vi "Execute.vi"(8 "error in":errorcluster, 11 "Filter STEP in":refnum<class "Filter STEP.lvclass">) -> (0 "error out":errorcluster, 1 "Next Step?":bool, 2 "MSG":string, 3 "Filter STEP out":refnum<class "Filter STEP.lvclass">)   [LabVIEW 2014, in "Filter STEP.lvclass"]
uses:
  Filter STEP.lvclass
  <vilib>/ActorFramework/Message Enqueuer/Message Enqueuer.lvclass
  Controller/Messages/Change Filter State/Change Filter State.lvclass
  Controller/Messages/Update Switch State MSG/Update Switch MSG.lvclass/Update Switch MSG.ctl
  <vilib>/ActorFramework/Message Enqueuer/Message Enqueuer.lvclass/Message Enqueuer.ctl
  Controller/Messages/Update Switch State MSG/Write Val.vi
  <vilib>/ActorFramework/Message Priority Queue/Priority Enqueue.vi
  c/exscalabar/steps/SEQ.lvlibp/STEPS/Read Obj.vi
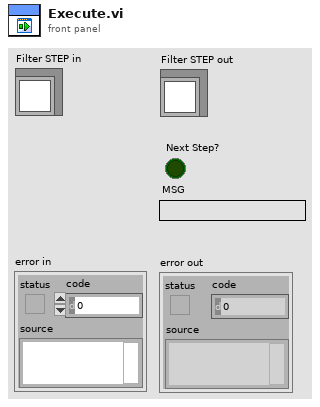
[diagram p1: front panel]
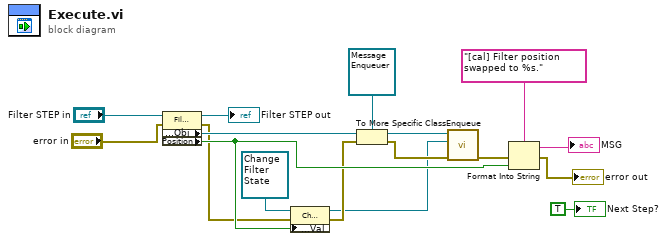
[diagram p0: block diagram]
diagram:
  n1 = property class="Filter"(reference="Filter STEP in", error in="error in") -> (reference out=→"Filter STEP out":refnum<class "Filter STEP.lvclass">, error out=w10:errorcluster, "Accessors:Obj"=w17:refnum<class>, "Position"=w11:bool)
  n2 = property class="Change Filter State MSG"(reference=refnum<class "Change Filter State.lvclass"> refnum ("Controller:Change Filter State MSG"), error in=w10, "Accessors:Val"=w11) -> (reference out=w2:refnum<class "Change Filter State.lvclass">, error out=w9:errorcluster)
  n3 = To More Specific Class(target class=refnum<class "Message Enqueuer.lvclass"> refnum ("Message Enqueuer in"), reference=w17, error in=w9) -> (specific class reference=w14:refnum<class "Message Enqueuer.lvclass">, error out=w15:errorcluster)
  n4 = call <vilib>:"Enqueue.vi"("error in (no error)"=w15, "Message"=w2, "Message Enqueuer in"=w14) -> ("error out"=w12:errorcluster)  [unwired: 7 in, 1 out]
  n5 = Format Into String(format string="[cal] Filter position swapped to %s.", error in=w12, w11) -> (resulting string=→"MSG":string, error out=→"error out":errorcluster)  [unwired: 1 in]
  "Next Step?" <- TRUE ("Next Step?")
